vi "XIPIN_AXI-Stream_FIFO_4_1.vi"   [LabVIEW 2017]
doc: "AXI-Stream FIFO converts memory mapped transactions to AXI-Stream transactions and vice versa. Choose desired data interface (AXI4 or AXI4-Lite), FIFO depth, Data width of AXI interface (data width of the interfaces are same) and cut-through mode or packet mode.\n------------------------------------\n<b>Need License</b> : No\n<b>Interface</b> : AXI4 AXI4-Stream"
uses:
  <vilib>/rvi/XilinxIP/XIPIN_XNode/niFpgaXIPIN.xnode
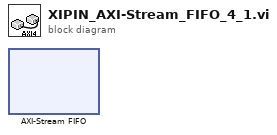
[diagram p0: block diagram]
diagram:
  n1 = xnode ("AXI-Stream FIFO")() -> ()
